vi "VoltageRatioInputGetSensorUnit.vi"(0 "error in (no error)":errorcluster, 3 "Device In":u64) -> (7 "error out":errorcluster, 8 "name":string, 9 "symbol":string, 10 "Device Out":u64)   [LabVIEW 2012, in "Phidget Voltage Ratio Input.lvlib"]
doc: "${SensorUnit:Header}"
uses:
  <instrlib>/Phidgets/Phidget Voltage Ratio Input/Phidget Voltage Ratio Input.lvlib
  <vilib>/Utility/importsl/GetValueByPointer/datatype.ctl
  <vilib>/Utility/importsl/GetValueByPointer/GetValueByPointer.xnode
  <instrlib>/Phidgets/Phidget Common/Phidget Common.lvlib
  phidget22.dll
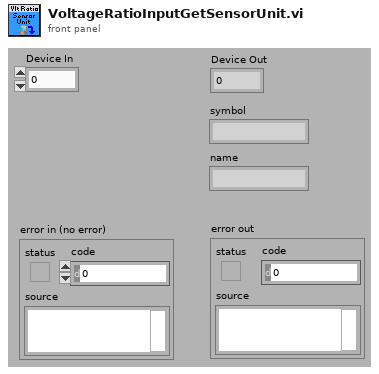
[diagram p1: front panel]
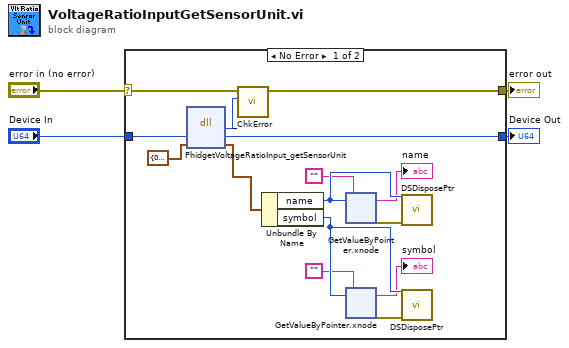
[diagram p0: block diagram]
diagram:
  n1 = case shown="No Error" "error in (no error)" {
    selector: "error in (no error)" -> [w16 w45]
    tunnel: [w15 w45] -> w3
    tunnel: "Device In" -> [w19 w44]
    tunnel: [w18 w44] -> w1
    frame No Error {
      n2 = dll-call lib="phidget22.*" fn="PhidgetVoltageRatioInput_getSensorUnit"("phid"=w19, "temperature"=cluster{"unit":u32, "name":u32, "symbol":u32} {"unit"=0, "name"=0, "symbol"=0} ("sensorUnit")) -> ("return type"=w17:i32, "phid"=w18:u64, "temperature"=w5:cluster{"unit":u32, "name":u32, "symbol":u32})  [unwired: 3 in, 2 out]
      n3 = call <instrlib>:"_ChkError.vi"("Return Code"=w17, "error in (no error)"=w16) -> ("error out"=w15:errorcluster)  [unwired: 9 in]
      n4 = Unbundle By Name(w5) -> ("name"=w13:u32, "symbol"=w9:u32)
      n5 = xnode "GetValueByPointer.xnode"("Pointer"=w13, "InputType"="") -> ("Output"=→"name":string, "ErrorOut"=w14:errorcluster)  [unwired: 2 in]
      n6 = xnode "GetValueByPointer.xnode"("Pointer"=w9, "InputType"="") -> ("Output"=→"symbol":string, "ErrorOut"=w10:errorcluster)  [unwired: 2 in]
      n7 = call <vilib>:"DSDisposePtr.vi"("error in (no error)"=w14, "Pointer"=w13) -> ()  [unwired: 9 in, 1 out]
      n8 = call <vilib>:"DSDisposePtr.vi"("error in (no error)"=w10, "Pointer"=w9) -> ()  [unwired: 9 in, 1 out]
    }
    frame Error {
    }
  }
  "error out" <- w3
  "Device Out" <- w1
